vi "SRV_Sensor PARSE_##R.vi"(0 "Return Data":string, 11 "error in (no error)":errorcluster) -> (3 "Sensor View Indicator Names":T1, 10 "Value":dbl, 15 "error out":errorcluster)   [LabVIEW 2014]
uses:
  SRV_Sensors Names.ctl
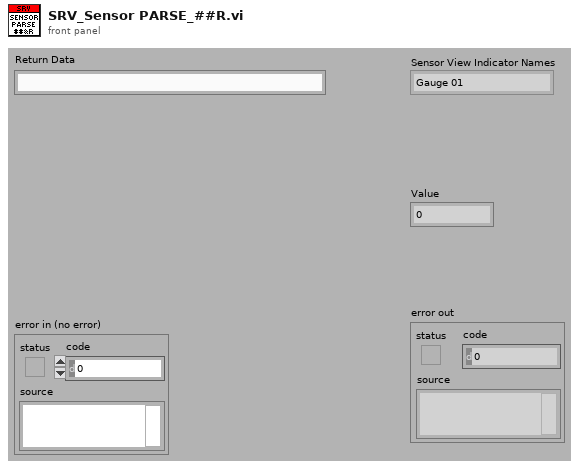
[diagram p1: front panel]
types:
  T1 = typedef "SRV_Sensors Names.ctl" = enum16{"Gauge 01", "Gauge 02", "Gauge 03", "Gauge 04", "Meter 01", "Meter 02", "Meter 03", "Meter 04", "Numeric 01", "Numeric 02", "Numeric 03", "Numeric 04", "Numeric 05", "Numeric 06", "Numeric 07", "Numeric 08", "Boolean 01", "Boolean 02", "Boolean 03", "Boolean 04", "Boolean 05", "Boolean 06", "Boolean 07", "Boolean 08", "Boolean 09", "Boolean 10", "Boolean 11", "Boolean 12", "Boolean 13", "Boolean 14", "Boolean 15", "Boolean 16", "Boolean 17", "Boolean 18", "Boolean 19", "Boolean 20", "Boolean 21", "Boolean 22", "Boolean 23", "Boolean 24", "Boolean 25", "Boolean 26", "Boolean 27", "Boolean 28", "Boolean 29", "Boolean 30", "Boolean 31", "Boolean 32"}
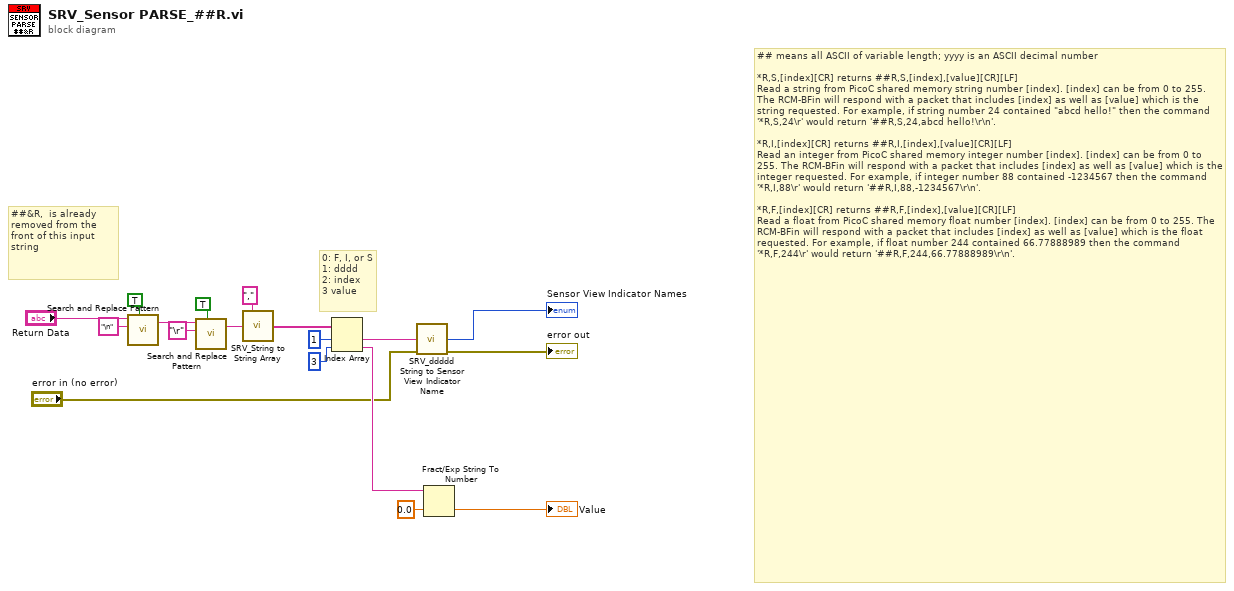
[diagram p0: block diagram]
diagram:
  # "0: F, I, or S\n1: dddd\n2: index\n3 value"
  # "##&R,  is already removed from the front of this input string"
  # "## means all ASCII of variable length; yyyy is an ASCII decimal number\n\n*R,S,[index][CR] returns ##R,S,[index],[value][CR][LF]\nRead a string from PicoC shared memory string number [index]. [index] can be from 0 to 255. The RCM-BFin will respond with a packet that includes [index] as well as [value] which is the string requested. For example, if string number 24 contained \"abcd hello!\" then the command '*R,S,24\\r' would return '##R,S,24,abcd hello!\\r\\n'.\n\n*R,I,[index][CR] returns ##R,I,[index],[value][CR][LF]\nRead an integer from PicoC shared memory integer number [index]. [index] can be from 0 to 255. The RCM-BFin will respond with a packet that includes [index] as well as [value] which is the integer requested. For example, if integer number 88 contained -1234567 then the command '*R,I,88\\r' would return '##R,I,88,-1234567\\r\\n'.\n\n*R,F,[index][CR] returns ##R,F,[index],[value][CR][LF]\nRead a float from PicoC shared memory float number [index]. [index] can be from 0 to 255. The RCM-BFin will respond with a packet that includes [index] as well as [value] which is the float requested. For example, if float number 244 contained 66.77888989 then the command '*R,F,244\\r' would return '##R,F,244,66.77888989\\r\\n'."
  n1 = call <vilib>:"Search and Replace Pattern.vi"("string"="Return Data", "regular expression (\"\")"="\n" ("regular expression (\"\")"), "replace all? (F)"=TRUE) -> ("result string"=w13:string)  [unwired: 2 in, 1 out]
  n2 = call <vilib>:"Search and Replace Pattern.vi"("string"=w13, "regular expression (\"\")"="\r" ("regular expression (\"\")"), "replace all? (F)"=TRUE) -> ("result string"=w12:string)  [unwired: 2 in, 1 out]
  n3 = call "SRV_String to String Array.vi"("Element Separator (,)"=",", "String"=w12) -> ("String Array"=w10:string[])  [unwired: 13 in]
  n4 = Index Array(array=w10, index #1=1 ("index"), index #2=3 ("index")) -> (element #1=w6:string, element #2=w3:string)
  n5 = call "SRV_ddddd String to Sensor View Indicator Name.vi"("ddddd"=w6, "error in (no error)"="error in (no error)") -> ("Sensor View Indicator Names"=→"Sensor View Indicator Names":T1, "error out"=→"error out":errorcluster)  [unwired: 12 in]
  n6 = Fract/Exp String To Number(string=w3, default (0 dbl)=0.0 ("default (0 DBL)")) -> (number=→"Value":dbl)  [unwired: 2 in, 1 out]
